vi "lab2(basic;works).vi"() -> ()   [LabVIEW 2016]
panel:
  out "2D Picture":picture
  in  "SwapGB":bool
  in  "SwapRB":bool
  in  "SwapRG":bool
  in  "Original":bool
  in  "ImagePath":path
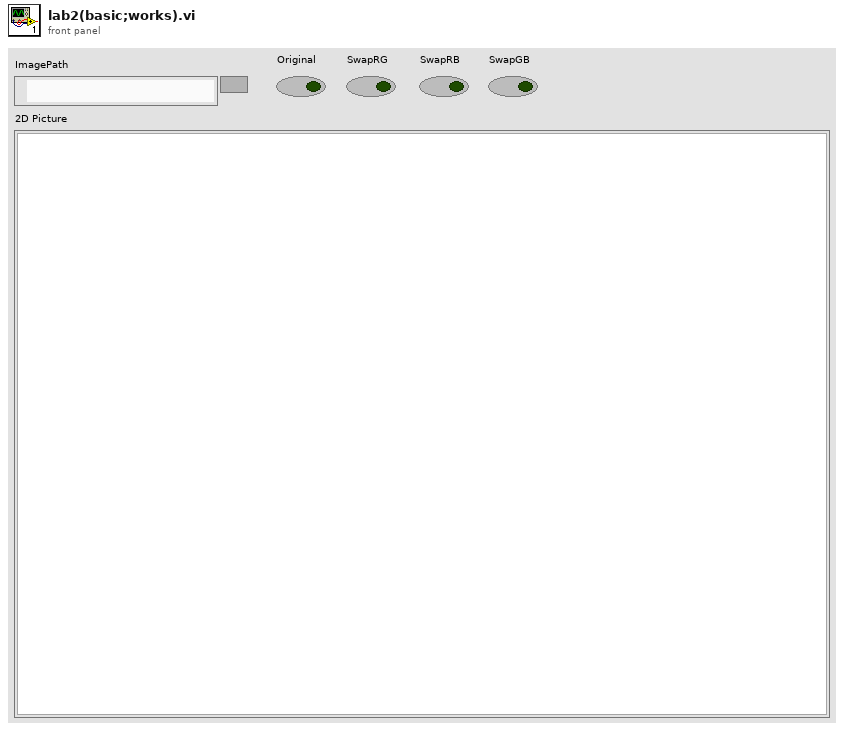
[diagram p1: front panel]
types:
  T1 = typedef "imagedata.ctl" = cluster{"image type":i32, "image depth":i32, "image":u8[], "mask":u8[], "colors":u32[], "Rectangle":cluster{"left":i16, "top":i16, "right":i16, "bottom":i16}}
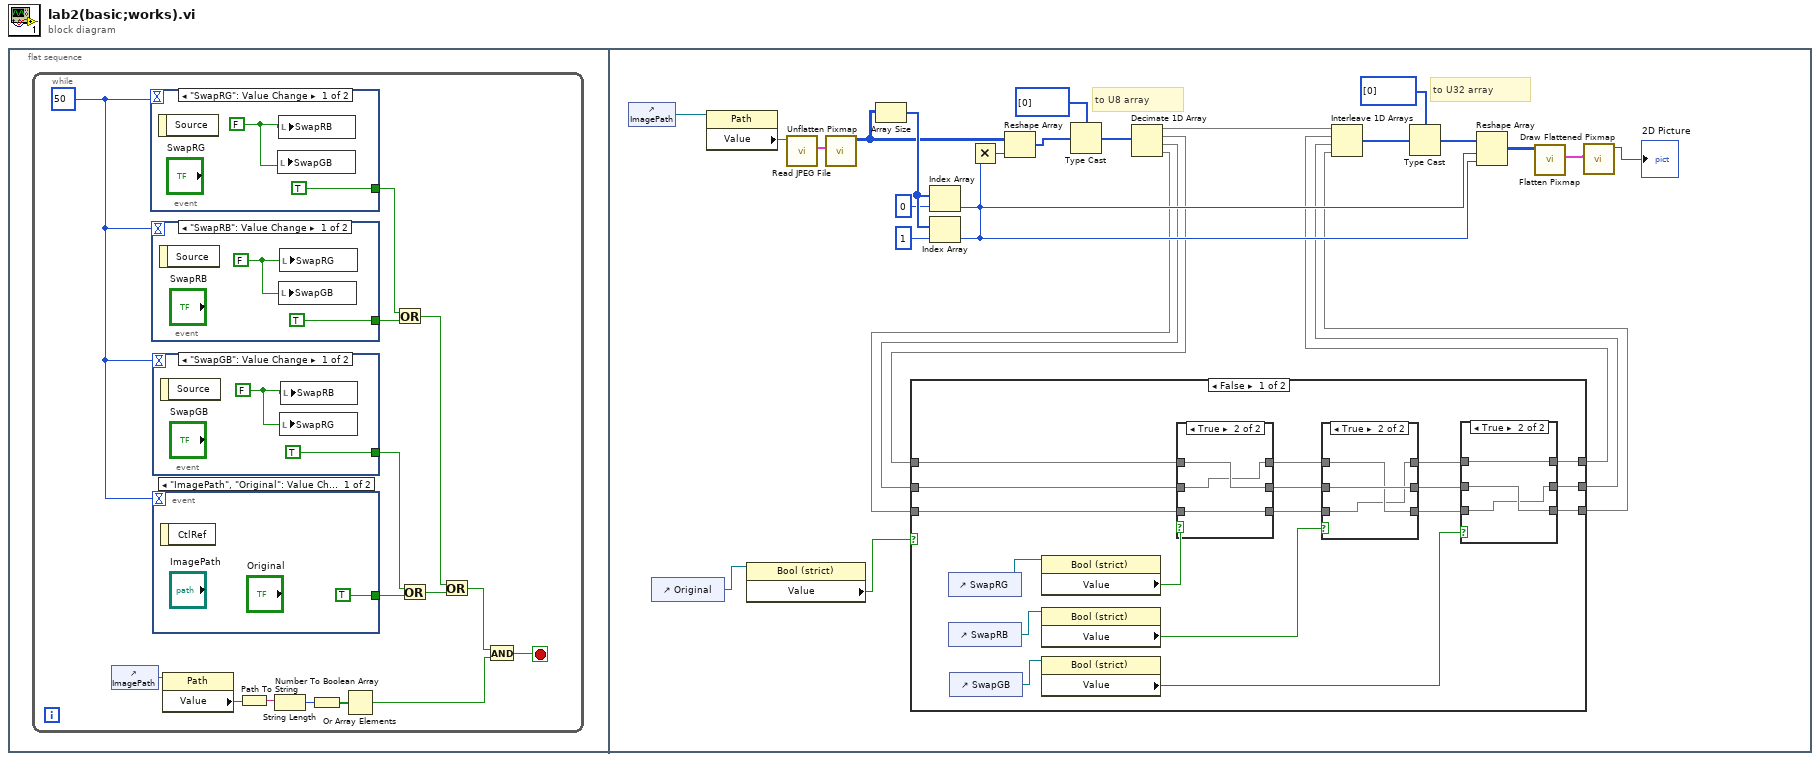
[diagram p0: block diagram]
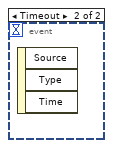
[diagram p2: hidden frame]
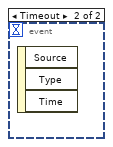
[diagram p3: hidden frame]
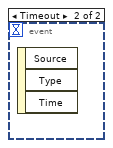
[diagram p4: hidden frame]
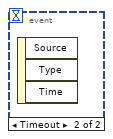
[diagram p5: hidden frame]
diagram:
  n1 = flat-sequence {
    frame #0 {
      n2 = while {
        stop <- w3 stop-if-true
        w11 = 50
        n3 = control-ref of="ImagePath"() -> (w15:refnum<vi>)
        n4 = event shown="[0] \"SwapRG\": Value Change" {
          selector: _ -> [_ _]
          dyn-events: _ -> [_ _]
          timeout: w11 -> [_ _]
          tunnel: [TRUE _] -> w5
          event "SwapRG": Value Change {
            w21 = FALSE
            n5 = event-data() -> ()  [unwired: 1 in, 1 out]
            n6 = local write "SwapGB"(w21) -> ()
            n7 = local write "SwapRB"(w21) -> ()
          }
          event Timeout {
            n8 = event-data() -> ()  [unwired: 1 in, 3 out]
          }
        }
        n9 = event shown="[0] \"SwapRB\": Value Change" {
          selector: _ -> [_ _]
          dyn-events: _ -> [_ _]
          timeout: w11 -> [_ _]
          tunnel: [TRUE _] -> w8
          event "SwapRB": Value Change {
            w19 = FALSE
            n10 = event-data() -> ()  [unwired: 1 in, 1 out]
            n11 = local write "SwapGB"(w19) -> ()
            n12 = local write "SwapRG"(w19) -> ()
          }
          event Timeout {
            n13 = event-data() -> ()  [unwired: 1 in, 3 out]
          }
        }
        n14 = event shown="[0] \"SwapGB\": Value Change" {
          selector: _ -> [_ _]
          dyn-events: _ -> [_ _]
          timeout: w11 -> [_ _]
          tunnel: [TRUE _] -> w4
          event "SwapGB": Value Change {
            w17 = FALSE
            n15 = event-data() -> ()  [unwired: 1 in, 1 out]
            n16 = local write "SwapRG"(w17) -> ()
            n17 = local write "SwapRB"(w17) -> ()
          }
          event Timeout {
            n18 = event-data() -> ()  [unwired: 1 in, 3 out]
          }
        }
        n19 = event shown="[0] \"ImagePath\", \"Original\": Value Change" {
          selector: _ -> [_ _]
          dyn-events: _ -> [_ _]
          timeout: w11 -> [_ _]
          tunnel: [TRUE _] -> w9
          event "ImagePath", "Original": Value Change {
            n20 = event-data() -> ()  [unwired: 1 in, 1 out]
          }
          event Timeout {
            n21 = event-data() -> ()  [unwired: 1 in, 3 out]
          }
        }
        n22 = property class="Path"(reference=w15) -> ("Value"=w14:path)  [unwired: 1 in, 2 out]
        n23 = Path To String(path=w14) -> (string=w13:string)
        n24 = String Length(string=w13) -> (length=w10:i32)
        n25 = Number To Boolean Array(number=w10) -> (Boolean array=w12:bool[])
        n26 = Or Array Elements(Boolean array=w12) -> (logical OR=w1:bool)
        n27 = Or(x=w5, y=w8) -> (x .or. y?=w6:bool)
        n28 = Or(x=w4, y=w9) -> (x .or. y?=w7:bool)
        n29 = Or(x=w6, y=w7) -> (x .or. y?=w2:bool)
        n30 = And(x=w2, y=w1) -> (x .and. y?=w3:bool)
      }
    }
    frame #1 {
      # "to U32 array"
      # "to U8 array"
      n31 = control-ref of="ImagePath"() -> (w38:refnum<vi>)
      n32 = control-ref of="Original"() -> (w30:refnum<vi>)
      n33 = property class="Path"(reference=w38) -> ("Value"=w39:path)  [unwired: 1 in, 2 out]
      n34 = property class="Bool (strict)"(reference=w30) -> ("Value"=w29:bool)  [unwired: 1 in, 2 out]
      n35 = call <vilib>:"Read JPEG File.vi"("path to JPEG file"=w39) -> ("image data"=w50:T1)  [unwired: 8 in, 2 out]
      n36 = call <vilib>:"Unflatten Pixmap.vi"("image data"=w50) -> ("24-bit pixmap"=w40:u32[][])  [unwired: 4 in, 6 out]
      n37 = Array Size(array=w40) -> (size(s)=w43:i32[])
      n38 = Index Array(array=w43, index=0) -> (element=w48:i32)
      n39 = Index Array(array=w43, index=1) -> (element=w49:i32)
      n40 = Multiply(x=w49, y=w48) -> (x*y=w47:i32)
      n41 = Reshape Array(w40, w47) -> (w34:u32[])
      n42 = Type Cast(type=u8[] [0], x=w34) -> (*(type *) &x=w33:u8[])
      n43 = Decimate 1D Array(w33) -> (w35:u8[], w28:u8[], w27:u8[], w26:u8[])
      n44 = case shown="False" w29 {
        tunnel: w28 -> [w56 w89]
        tunnel: w27 -> [w55 w88]
        tunnel: w26 -> [w54 w87]
        tunnel: [w53 w89] -> w25
        tunnel: [w52 w88] -> w24
        tunnel: [w51 w87] -> w23
        frame False {
          n45 = control-ref of="SwapRG"() -> (w68:refnum<vi>)
          n46 = control-ref of="SwapRB"() -> (w60:refnum<vi>)
          n47 = control-ref of="SwapGB"() -> (w58:refnum<vi>)
          n48 = property class="Bool (strict)"(reference=w68) -> ("Value"=w67:bool)  [unwired: 1 in, 2 out]
          n49 = property class="Bool (strict)"(reference=w60) -> ("Value"=w59:bool)  [unwired: 1 in, 2 out]
          n50 = property class="Bool (strict)"(reference=w58) -> ("Value"=w57:bool)  [unwired: 1 in, 2 out]
          n51 = case shown="True" w67 {
            tunnel: w54 -> [w83 w84]
            tunnel: w55 -> [w82 w85]
            tunnel: w56 -> [w81 w86]
            tunnel: [w83 w84] -> w63
            tunnel: [w82 w86] -> w64
            tunnel: [w81 w85] -> w66
            frame False {
            }
            frame True {
            }
          }
          n52 = case shown="True" w59 {
            tunnel: w63 -> [w77 w78]
            tunnel: w64 -> [w76 w80]
            tunnel: w66 -> [w75 w79]
            tunnel: [w77 w79] -> w61
            tunnel: [w76 w80] -> w62
            tunnel: [w75 w78] -> w65
            frame False {
            }
            frame True {
            }
          }
          n53 = case shown="True" w57 {
            tunnel: w61 -> [w71 w72]
            tunnel: w62 -> [w70 w73]
            tunnel: w65 -> [w69 w74]
            tunnel: [w71 w73] -> w51
            tunnel: [w70 w72] -> w52
            tunnel: [w69 w74] -> w53
            frame False {
            }
            frame True {
            }
          }
        }
        frame True {
        }
      }
      n54 = Interleave 1D Arrays(w35, w25, w24, w23) -> (w32:u8[])
      n55 = Type Cast(type=u32[] [0], x=w32) -> (*(type *) &x=w31:u32[])
      n56 = Reshape Array(w31, w48, w49) -> (w44:u32[][])
      n57 = call <vilib>:"Flatten Pixmap.vi"("24-bit pixmap"=w44) -> ("image data"=w45:T1)  [unwired: 10 in]
      n58 = call <vilib>:"Draw Flattened Pixmap.vi"("image data"=w45) -> ("new picture"=→"2D Picture":picture)  [unwired: 8 in]
    }
  }
